vi "Create Stream Content.vi"(5 "HttpContent_Stream in":refnum<class "HttpContent_Stream.lvclass">, 8 "error in (no error)":errorcluster, 11 "content":refnum<k24>) -> (0 "error out":errorcluster, 3 "HttpContent_Stream out":refnum<class "HttpContent_Stream.lvclass">)   [LabVIEW 2018, in "LabVIEWHTTPClient_NET.lvlib" / "HttpContent_Stream.lvclass"]
uses:
  HttpContent_Stream.lvclass
  C:/Viviota/Projects/R&D/LabVIEW_HTTP_REST_NET/HttpContent/HttpContent.lvclass
  System.Net.Http
  HttpContent/HttpContent.lvclass
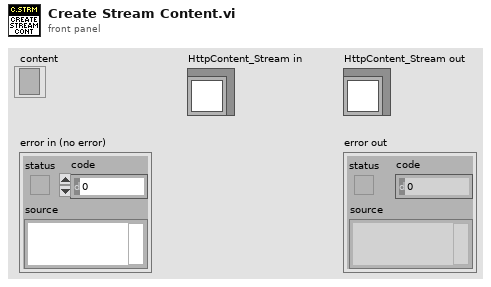
[diagram p1: front panel]
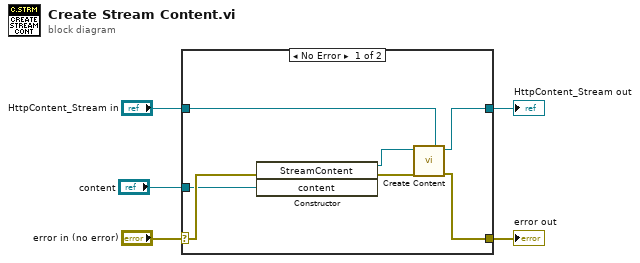
[diagram p0: block diagram]
diagram:
  n1 = case shown="No Error" "error in (no error)" {
    selector: "error in (no error)" -> [w8 w14]
    tunnel: [w6 w14] -> w4
    tunnel: [w9 w13] -> w2
    tunnel: "HttpContent_Stream in" -> [w10 w13]
    tunnel: "content" -> [w7 _]
    frame No Error {
      n2 = constructor class="StreamContent"(error in=w8, "content"=w7) -> (reference out=w11:refnum<k24>, error out=w12:errorcluster)  [unwired: 2 in, 2 out]
      n3 = call "Create Content.vi"("HttpContent in"=w10, "error in (no error)"=w12, "NET_HttpContent"=w11) -> ("error out"=w6:errorcluster, "HttpContent out"=w9:refnum<class "HttpContent_Stream.lvclass">)  [unwired: 7 in]
    }
    frame Error {
    }
  }
  "error out" <- w4
  "HttpContent_Stream out" <- w2
